vi "sub_gpxfile-2-latlong.vi"(11 "wpt Array":string[][](array[string])) -> (3 "배열":cluster{dbl, dbl}[](array[cluster]))   [LabVIEW 2019]
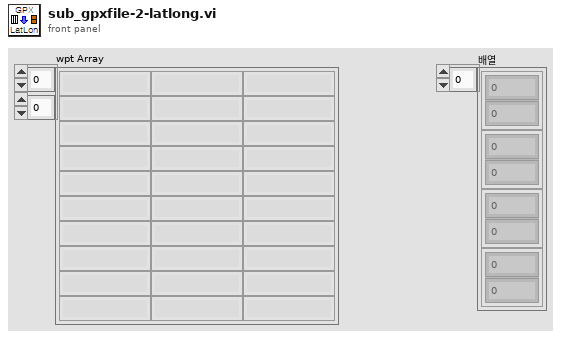
[diagram p1: front panel]
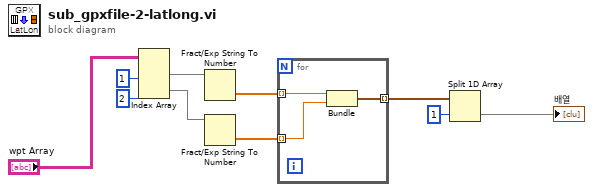
[diagram p0: block diagram]
diagram:
  n1 = Index Array(array="wpt Array", index (col) #1=1 ("비활성화된 인덱스 (열)"), index (col) #2=2 ("인덱스 (열)")) -> (element #1=w6:string[], element #2=w4:string[])  [unwired: 2 in]
  n2 = Fract/Exp String To Number(string=w6) -> (number=w5:dbl[])  [unwired: 3 in, 1 out]
  n3 = Fract/Exp String To Number(string=w4) -> (number=w7:dbl[])  [unwired: 3 in, 1 out]
  n4 = for {
    tunnel: w5 -> [w13] mode=indexing
    tunnel: w7 -> [w12] mode=indexing
    tunnel: [w11] -> w8 mode=indexing
    n5 = Bundle(w13, w12) -> (w11:cluster{dbl, dbl})  [unwired: 1 in]
  }
  n6 = Split 1D Array(array=w8, index=1 ("인덱스")) -> (second subarray=→"배열":cluster{dbl, dbl}[])  [unwired: 1 out]
